vi "Preprocess Action.vi"(0 "Image Type":T2 items=["Grayscale (U8)", "Grayscale (I16)", "Grayscale (SGL)", "Complex (CSG)", "RGB (U32)", "HSL (U32)", "RGB (U64)", "Grayscale (U16)"], 1 "Image Dust":string, 5 "ImageSorce":string, 9 "PreProcess":T1, 11 "error in (no error)":errorcluster, 12 "Data":string) -> (4 "Refnum out":T3, 15 "error out":errorcluster)   [LabVIEW 2019]
uses:
  <vilib>/vision/Image Controls.llb/IMAQ Image.ctl
  Ctrl/VisionProcessName.ctl
  Controls/Process_Setting.ctl
  Controls/CameraAttribute.ctl
  Controls/ProcessBrightness.ctl
  Controls/ExtractPlanParam_Type.ctl
  Controls/ProcessColorThreshold.ctl
  Controls/LookupTableParam.ctl
  Controls/BinaryMonoParam_Type.ctl
  7215dd0e-a700-4e2b-943e-45d7582282bd.vi
  38a9804b-11bb-4e90-8cf5-6f7932444913.vi
  4fbe3eb4-3ab0-49f8-8326-0d8c4c82d423.vi
  17e7e0cf-ffba-40d4-8f93-2ae686572284.vi
  f6032967-3aff-41e1-8fb3-f70b6d7b46ba.vi
  79f2a73c-968e-4675-82f3-10344eb773ba.vi
  0b9d5edb-3a18-4d09-8481-e8059829d2ca.vi
  <vilib>/JDP Science/JSONtext/JSON text to Variant.vi
  <resource>/objmgr/imaqdx.rc
  LLB/Message/MsgShowAndLog.lvlib
panel:
  in  "AutoExposure":enum16{"Off", "Once", "Continuous"}(ring)
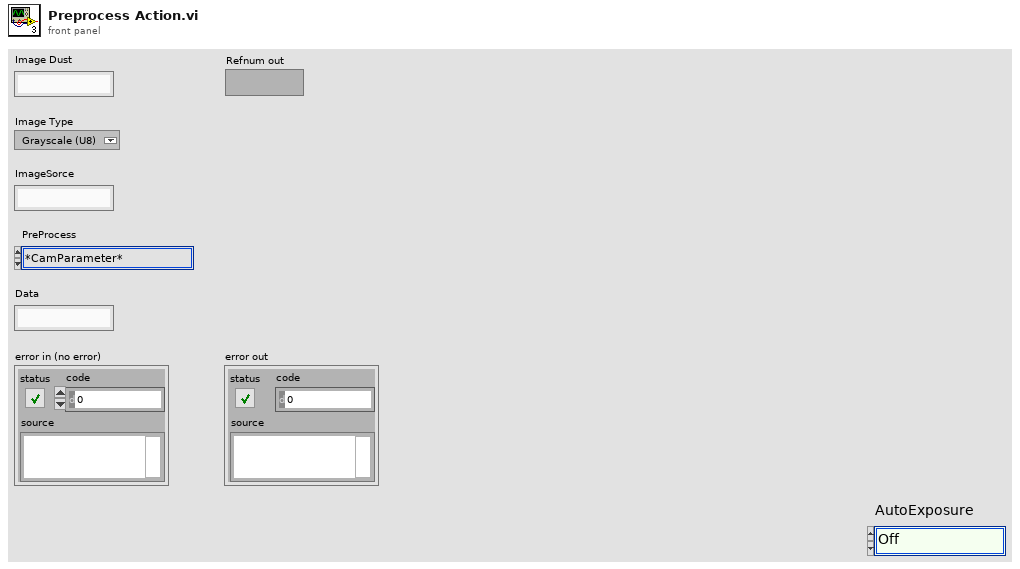
[diagram p1: front panel]
types:
  T1 = typedef "VisionProcessName.ctl" = enum16{"*CamParameter*", "CamAttributes", "*Preprocess*", "CG_Brightness", "C_Plane Extraction", "C_Threshold", "G_Lookup Table", "G_Threshold"}
  T2 = typedef "Image Type" = u32
  T3 = typedef "IMAQ Image.ctl" = refnum<image>
  T4 = typedef "Process_Setting.ctl" = cluster{"Enum_PreProcess":T1, "Parameter":string}
  T5 = enum16{"Init", "Grab", "Get All", "Close", "Set Camera"}
  T6 = typedef "CameraAttribute.ctl" = cluster{"CamName":string, "AutoExposure":enum16{"Off", "Once", "Continuous"}, "Exposure":dbl, "AutoGain":enum16{"Off", "Once", "Continuous"}, "Gain":dbl}
  T7 = typedef "BinaryMonoParam_Type.ctl" = cluster{"Look For":enum16{"Bright Objects", "Dark Objects", "Gray Objects"}, "Threshold":cluster{dbl, dbl}}
  T8 = typedef "IMAQdx.ctl" = refnum<k21>
  T9 = typedef "ProcessBrightness.ctl" = cluster{"Brightness":i32, "Constrast":dbl, "Gamma":dbl}
  T10 = typedef "ExtractPlanParam_Type.ctl" = cluster{"Color Plane":enum16{"Red", "Green", "Blue", "Hue", "Saturation", "Luminance", "Value", "Intensity"}}
  T11 = enum16{"Red", "Green", "Blue", "Hue", "Saturation", "Luminance", "Value", "Intensity"}
  T12 = typedef "ProcessColorThreshold.ctl" = cluster{"Color Mode":u16, "Red or Hue Range":cluster{dbl, dbl}, "Green or Sat Range":cluster{dbl, dbl}, "Blue or Luma or Val or Inten Range":cluster{dbl, dbl}}
  T13 = typedef "LookupTableParam.ctl" = cluster{"Function":enum16{"Equalizer", "Reverse", "Logarithmic", "Exponential", "Square", "Square Root", "Power X", "Power 1/X"}, "Power Value":sgl}
  T14 = enum16{"Equalizer", "Reverse", "Logarithmic", "Exponential", "Square", "Square Root", "Power X", "Power 1/X"}
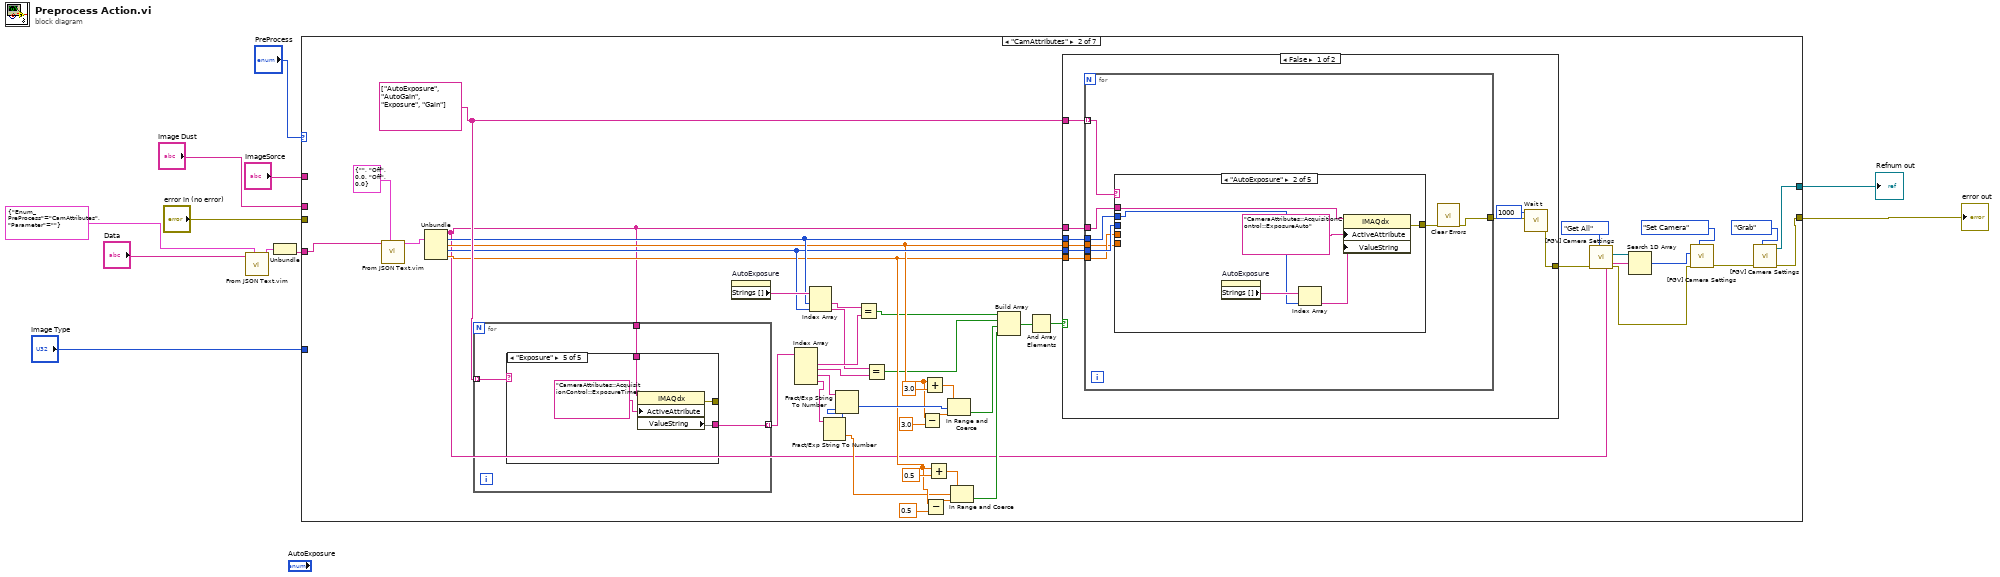
[diagram p0: block diagram]
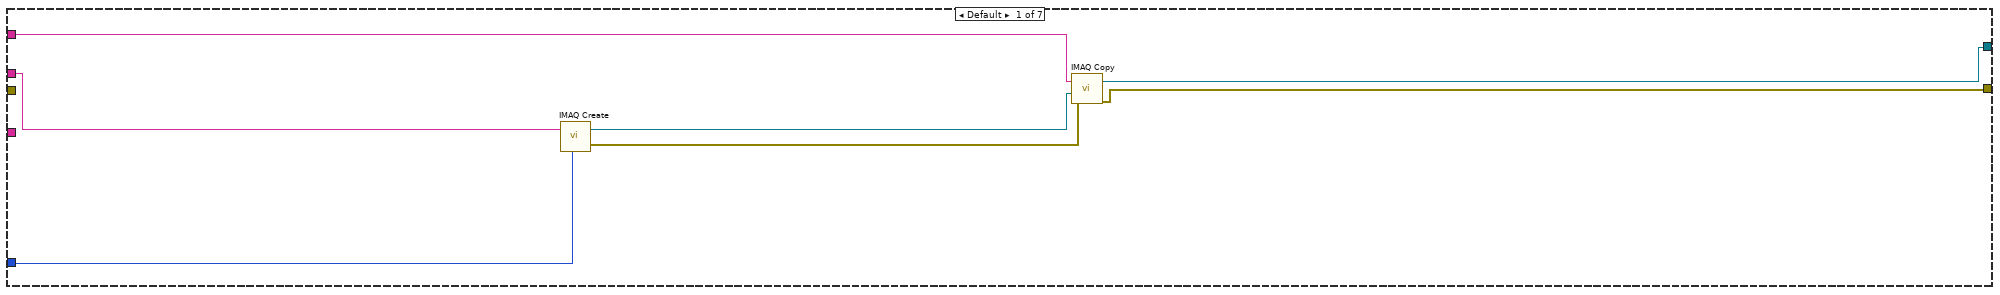
[diagram p2: hidden frame]
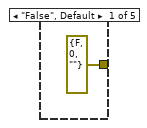
[diagram p3: hidden frame]
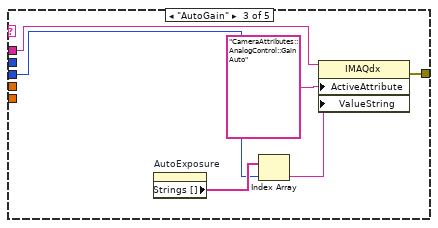
[diagram p4: hidden frame]
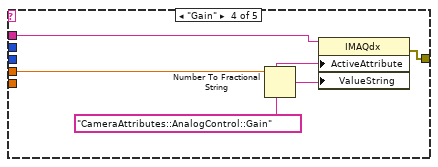
[diagram p5: hidden frame]
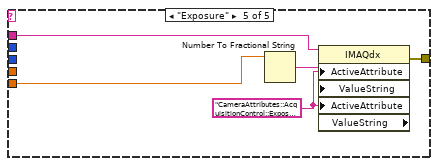
[diagram p6: hidden frame]
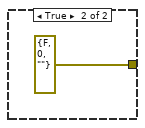
[diagram p7: hidden frame]
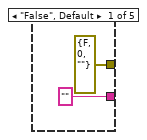
[diagram p8: hidden frame]
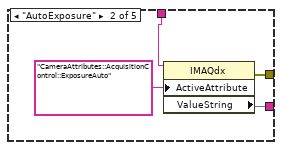
[diagram p9: hidden frame]
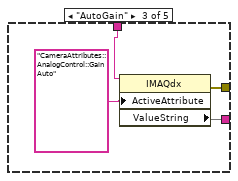
[diagram p10: hidden frame]
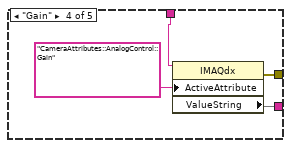
[diagram p11: hidden frame]
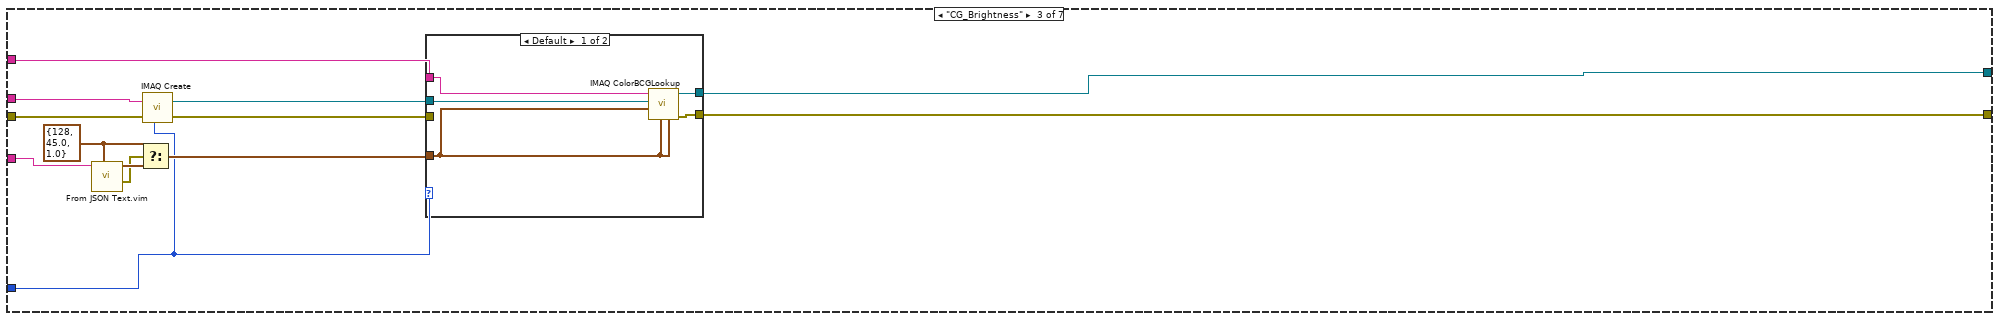
[diagram p12: hidden frame]
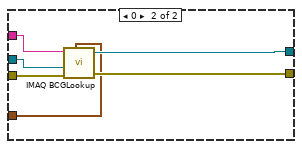
[diagram p13: hidden frame]
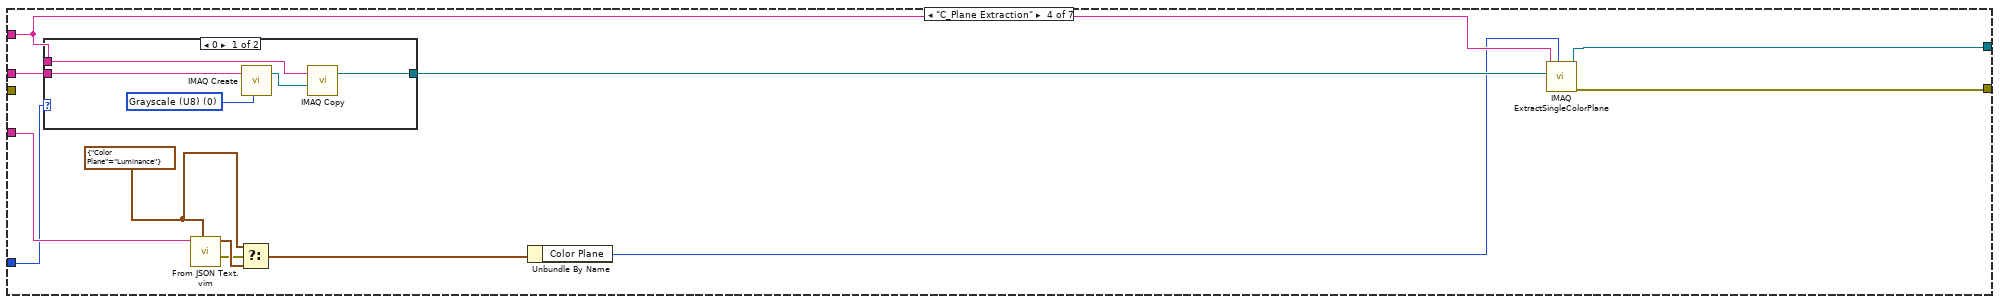
[diagram p14: hidden frame]
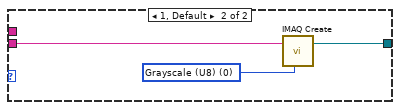
[diagram p15: hidden frame]
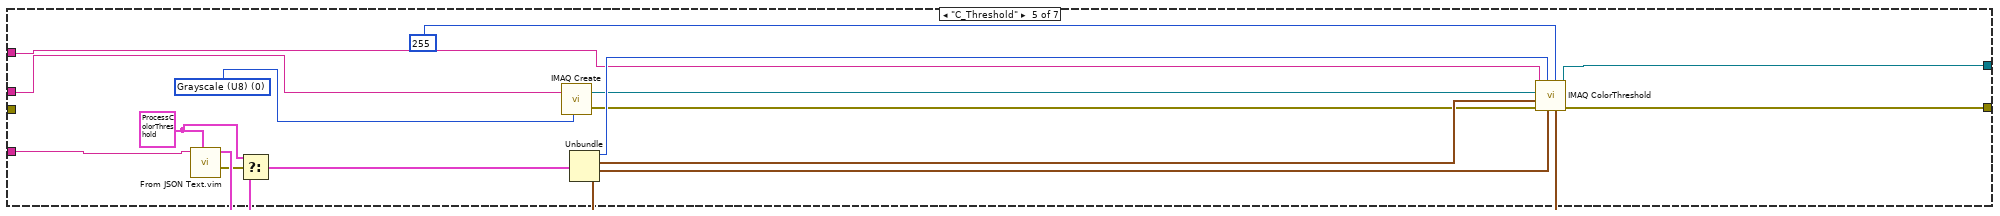
[diagram p16: hidden frame]
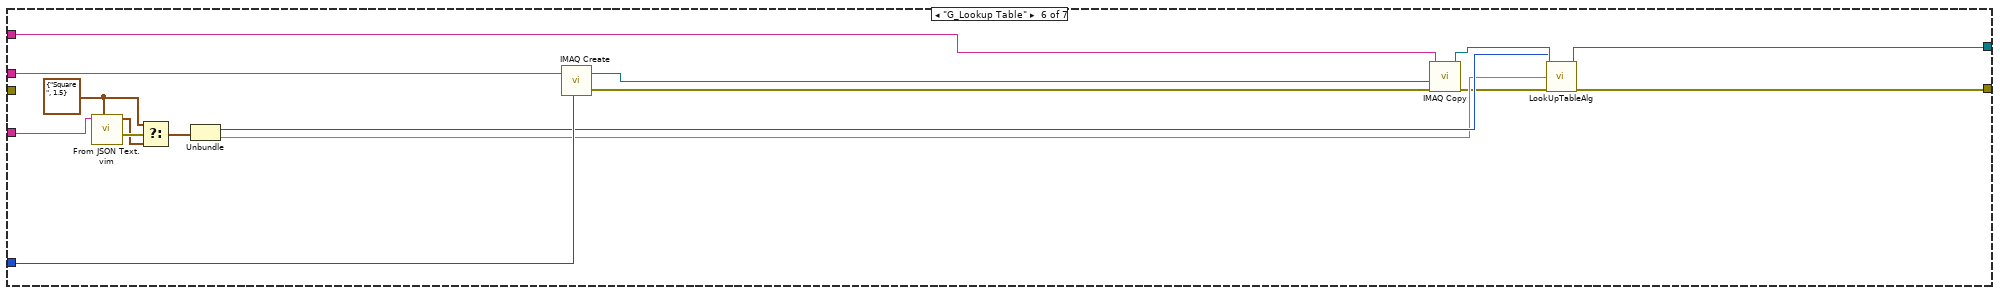
[diagram p17: hidden frame]
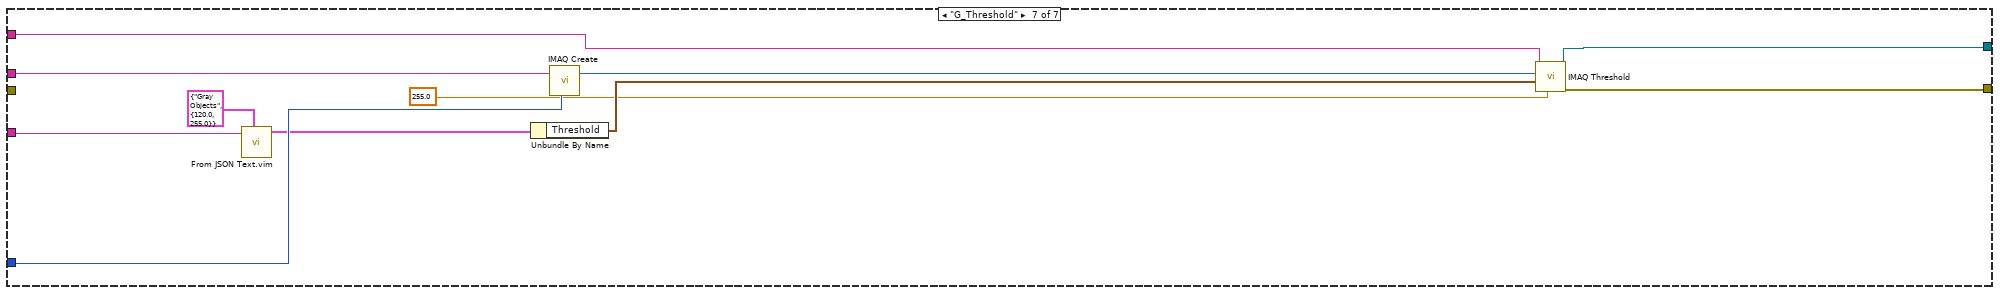
[diagram p18: hidden frame]
diagram:
  n1 = call "From JSON Text.vim"("Data Type and Default Value"=T4 {"Enum_PreProcess"=enum."CamAttributes", "Parameter"=""} ("ProcessSetting"), "JSON"="Data") -> ("Data out"=w3:T4)  [unwired: 8 in, 1 out]
  n2 = Unbundle(w3) -> ("Parameter"=w2:string)  [unwired: 1 out]
  n3 = case shown="\"CamAttributes\"" "PreProcess" {
    tunnel: "Image Type" -> [w18 _ w125 w156 _ w200 w209]
    tunnel: "error in (no error)" -> [_ _ w137 _ _ _ _]
    tunnel: "Image Dust" -> [w17 _ w136 w155 w181 w201 w211]
    tunnel: [w14 w50 w135 w149 w174 w192 w204] -> w9
    tunnel: [w13 w51 w133 w150 w173 w193 w203] -> w10
    tunnel: w2 -> [_ w60 w129 w157 w182 w190 w210]
    tunnel: "ImageSorce" -> [w16 _ w126 w154 w171 w199 w208]
    frame Default {
      n4 = call "IMAQ Create"("Image Name"=w17, "Image Type"=w18) -> ("New Image"=w15:T3, "error out"=w12:errorcluster)  [unwired: 3 in]
      n5 = call "IMAQ Copy"("error in (no error)"=w12, "Image Dst"=w15, "Image Src"=w16) -> ("error out"=w13:errorcluster, "Image Dst Out"=w14:T3)  [unwired: 3 in]
    }
    frame "CamAttributes" {
      w49 = string[] ["AutoExposure", "AutoGain", "Exposure", "Gain"]
      n6 = call "From JSON Text.vim"("Data Type and Default Value"=T6 {"CamName"="", "AutoExposure"=enum."Off", "Exposure"=0.0, "AutoGain"=enum."Off", "Gain"=0.0} ("CamAttribute"), "JSON"=w60) -> ("Data out"=w61:T6)  [unwired: 8 in, 1 out]
      n7 = Unbundle(w61) -> ("CamName"=w21:string, "AutoExposure"=w47:enum16{"Off", "Once", "Continuous"}, "Exposure"=w37:dbl, "AutoGain"=w46:enum16{"Off", "Once", "Continuous"}, "Gain"=w31:dbl)
      n8 = for {
        tunnel: w49 -> [w106] mode=indexing
        tunnel: [w105] -> w44 mode=indexing
        tunnel: w21 -> [w104]
        n9 = case shown="\"Exposure\"" w106 {
          tunnel: [errorcluster {"status"=FALSE, "code"=0, "source"=""} ("error out") w111 w115 w119 w123] -> _
          tunnel: ["" ("ValueString") w110 w114 w118 w122] -> w105
          tunnel: w104 -> [_ w109 w113 w117 w121]
          frame "False", Default {
          }
          frame "AutoExposure" {
            n10 = property class="IMAQdx"(reference=w109, "ActiveAttribute"="CameraAttributes::AcquisitionControl::ExposureAuto") -> (error out=w111:errorcluster, "ValueString"=w110)  [unwired: 1 in, 1 out]
          }
          frame "AutoGain" {
            n11 = property class="IMAQdx"(reference=w113, "ActiveAttribute"="CameraAttributes::AnalogControl::GainAuto") -> (error out=w115:errorcluster, "ValueString"=w114)  [unwired: 1 in, 1 out]
          }
          frame "Gain" {
            n12 = property class="IMAQdx"(reference=w117, "ActiveAttribute"="CameraAttributes::AnalogControl::Gain") -> (error out=w119:errorcluster, "ValueString"=w118)  [unwired: 1 in, 1 out]
          }
          frame "Exposure" {
            n13 = property class="IMAQdx"(reference=w121, "ActiveAttribute"="CameraAttributes::AcquisitionControl::ExposureTime") -> (error out=w123:errorcluster, "ValueString"=w122)  [unwired: 1 in, 1 out]
          }
        }
      }
      n14 = property on="AutoExposure" class="Enum (strict)"() -> ("Strings []"=w48:string[])  [unwired: 2 in, 2 out]
      n15 = Index Array(array=w44) -> (element #1=w43:string, element #2=w20:string, element #3=w19:string, element #4=w29:string)  [unwired: 4 in]
      n16 = Index Array(array=w48, index #1=w47, index #2=w46) -> (element #1=w45:string, element #2=w42:string)
      n17 = Fract/Exp String To Number(string=w29) -> (offset past number=w30:i32, number=w28:dbl)  [unwired: 3 in]
      n18 = Fract/Exp String To Number(string=w19, default (0 dbl)=w30) -> (number=w41:i32)  [unwired: 2 in, 1 out]
      n19 = Equal?(x=w45, y=w43) -> (x = y?=w27:bool)
      n20 = Equal?(x=w42, y=w20) -> (x = y?=w26:bool)
      n21 = Subtract(x=w37, y=3.0) -> (x-y=w38:dbl)
      n22 = Add(x=w37, y=3.0) -> (x+y=w40:dbl)
      n23 = Subtract(x=w31, y=0.5) -> (x-y=w34:dbl)
      n24 = Add(x=w31, y=0.5) -> (x+y=w32:dbl)
      n25 = In Range and Coerce(upper limit=w40, x=w41, lower limit=w38) -> (In Range?=w25:bool)  [unwired: 1 out]
      n26 = In Range and Coerce(upper limit=w32, x=w28, lower limit=w34) -> (In Range?=w24:bool)  [unwired: 1 out]
      n27 = Build Array(w27, w26, w25, w24) -> (w23:bool[])
      n28 = And Array Elements(Boolean array=w23) -> (logical AND=w22:bool)
      n29 = case shown="False" w22 {
        tunnel: w21 -> [w71 _]
        tunnel: [w64 errorcluster {"status"=FALSE, "code"=0, "source"=""} ("error out")] -> w52
        tunnel: w49 -> [w69 _]
        tunnel: w47 -> [w68 _]
        tunnel: w46 -> [w67 _]
        tunnel: w37 -> [w66 _]
        tunnel: w31 -> [w65 _]
        frame False {
          n30 = for {
            tunnel: w69 -> [w72] mode=indexing
            tunnel: w68 -> [w79]
            tunnel: w71 -> [w78]
            tunnel: [w75] -> w70
            tunnel: w67 -> [w77]
            tunnel: w65 -> [w74]
            tunnel: w66 -> [w73]
            n31 = case shown="\"AutoExposure\"" w72 {
              tunnel: w79 -> [_ w84 _ _ _]
              tunnel: w78 -> [_ w83 w91 w93 w100]
              tunnel: w77 -> [_ _ w89 _ _]
              tunnel: [errorcluster {"status"=FALSE, "code"=0, "source"=""} ("error out") w81 w87 w94 w98] -> w76
              tunnel: w74 -> [_ _ _ w95 _]
              tunnel: w73 -> [_ _ _ _ w99]
              frame "False", Default {
              }
              frame "AutoExposure" {
                n32 = property on="AutoExposure" class="Enum (strict)"() -> ("Strings []"=w85:string[])  [unwired: 2 in, 2 out]
                n33 = Index Array(array=w85, index=w84) -> (element=w82:string)
                n34 = property class="IMAQdx"(reference=w83, "ActiveAttribute"="CameraAttributes::AcquisitionControl::ExposureAuto", "ValueString"=w82) -> (error out=w81:errorcluster)  [unwired: 1 in, 1 out]
              }
              frame "AutoGain" {
                n35 = property on="AutoExposure" class="Enum (strict)"() -> ("Strings []"=w90:string[])  [unwired: 2 in, 2 out]
                n36 = Index Array(array=w90, index=w89) -> (element=w88:string)
                n37 = property class="IMAQdx"(reference=w91, "ActiveAttribute"="CameraAttributes::AnalogControl::GainAuto", "ValueString"=w88) -> (error out=w87:errorcluster)  [unwired: 1 in, 1 out]
              }
              frame "Gain" {
                n38 = Number To Fractional String(number=w95) -> (F-format string=w96:string)  [unwired: 3 in]
                n39 = property class="IMAQdx"(reference=w93, "ActiveAttribute"="CameraAttributes::AnalogControl::Gain", "ValueString"=w96) -> (error out=w94:errorcluster)  [unwired: 1 in, 1 out]
              }
              frame "Exposure" {
                w102 = "CameraAttributes::AcquisitionControl::ExposureTime" ("ActiveAttribute")
                n40 = Number To Fractional String(number=w99) -> (F-format string=w101:string)  [unwired: 3 in]
                n41 = property class="IMAQdx" props=["ActiveAttribute", "ValueString", "ActiveAttribute", "ValueString"](reference=w100, "ActiveAttribute"=w102, "ValueString"=w101, "ActiveAttribute"=w102) -> (error out=w98:errorcluster)  [unwired: 1 in, 2 out]
              }
            }
            n42 = call <vilib>:"Clear Errors.vi"("error in (no error)"=w76) -> ("error out"=w75:errorcluster)  [unwired: 5 in, 1 out]
          }
          n43 = call "Wait t.vi"("error in"=w70, "wait(ms)"=u32 1000) -> ("error out"=w64:errorcluster)  [unwired: 9 in]
        }
        frame True {
        }
      }
      n44 = call "[FGV] Camera Settings.vi"("Action"=T5."Get All", "error in (no error)"=w52) -> ("error out"=w55:errorcluster, "Camera Interface Name"=w58:T8[])  [unwired: 7 in, 1 out]
      n45 = Search 1D Array(1D array=w58, element=w21) -> (index of element=w56:i32)  [unwired: 1 in]
      n46 = call "[FGV] Camera Settings.vi"("Action"=T5."Set Camera", "error in (no error)"=w55, "Value"=w56) -> ("error out"=w53:errorcluster)  [unwired: 6 in, 2 out]
      n47 = call "[FGV] Camera Settings.vi"("Action"=T5."Grab", "error in (no error)"=w53) -> ("error out"=w51:errorcluster, "Image Out"=w50:T3)  [unwired: 7 in, 1 out]
    }
    frame "CG_Brightness" {
      w132 = T9 {"Brightness"=128, "Constrast"=45.0, "Gamma"=1.0} ("t")
      n48 = call "From JSON Text.vim"("Data Type and Default Value"=w132, "JSON"=w129) -> ("error out"=w130:errorcluster, "Data out"=w131:T9)  [unwired: 8 in]
      n49 = Select(t=w132, s=w130, f=w131) -> (s? t:f=w128:T9)
      n50 = call "IMAQ Create"("Image Name"=w136, "Image Type"=w125, "error in (no error)"=w137) -> ("New Image"=w127:T3, "error out"=w134:errorcluster)  [unwired: 2 in]
      n51 = case shown="Default" w125 {
        tunnel: [w138 w148] -> w135
        tunnel: w134 -> [_ w147]
        tunnel: [w139 w146] -> w133
        tunnel: w128 -> [w140 w145]
        tunnel: w127 -> [w141 w144]
        tunnel: w126 -> [w142 w143]
        frame Default {
          n52 = call "IMAQ ColorBCGLookup"("Blue BCG Values"=w140, "Green BCG Values"=w140, "Red BCG Values"=w140, "Image Dst"=w141, "Image Src"=w142) -> ("error out"=w139:errorcluster, "Image Dst Out"=w138:T3)  [unwired: 2 in, 3 out]
        }
        frame 0 {
          n53 = call "IMAQ BCGLookup"("Image Src"=w143, "BCG Values"=w145, "Image Dst"=w144, "error in (no error)"=w147) -> ("Image Dst Out"=w148:T3, "error out"=w146:errorcluster)  [unwired: 1 in, 2 out]
        }
      }
    }
    frame "C_Plane Extraction" {
      w160 = T10 {"Color Plane"=enum."Luminance"} ("ExtractPlanParam")
      n54 = case shown="0" w156 {
        tunnel: w155 -> [w165 w168]
        tunnel: w154 -> [w162 _]
        tunnel: [w161 w166] -> w153
        frame 0 {
          w164 = T2 0 items=["Grayscale (U8)", "Grayscale (I16)", "Grayscale (SGL)", "Complex (CSG)", "RGB (U32)", "HSL (U32)", "RGB (U64)", "Grayscale (U16)"] ("Image Type")
          n55 = call "IMAQ Create"("Image Name"=w165, "Image Type"=w164) -> ("New Image"=w163:T3)  [unwired: 3 in, 1 out]
          n56 = call "IMAQ Copy"("Image Dst"=w163, "Image Src"=w162) -> ("Image Dst Out"=w161:T3)  [unwired: 4 in, 1 out]
        }
        frame 1, Default {
          w167 = T2 0 items=["Grayscale (U8)", "Grayscale (I16)", "Grayscale (SGL)", "Complex (CSG)", "RGB (U32)", "HSL (U32)", "RGB (U64)", "Grayscale (U16)"] ("Image Type")
          n57 = call "IMAQ Create"("Image Name"=w168, "Image Type"=w167) -> ("New Image"=w166:T3)  [unwired: 3 in, 1 out]
        }
      }
      n58 = call "From JSON Text.vim"("Data Type and Default Value"=w160, "JSON"=w157) -> ("error out"=w158:errorcluster, "Data out"=w159:T10)  [unwired: 8 in]
      n59 = Select(t=w160, s=w158, f=w159) -> (s? t:f=w152:T10)
      n60 = Unbundle By Name(w152) -> ("Color Plane"=w151:T11)
      n61 = call "IMAQ ExtractSingleColorPlane"("Color Plane"=w151, "Image Dst"=w153, "Image Src"=w154) -> ("error out"=w150:errorcluster, "Image Dst Out"=w149:T3)  [unwired: 7 in]
    }
    frame "C_Threshold" {
      w169 = T2 0 items=["Grayscale (U8)", "Grayscale (I16)", "Grayscale (SGL)", "Complex (CSG)", "RGB (U32)", "HSL (U32)", "RGB (U64)", "Grayscale (U16)"] ("Image Type")
      w184 = T12 {"Color Mode"=0, "Red or Hue Range"={120.0, 255.0}, "Green or Sat Range"={120.0, 255.0}, "Blue or Luma or Val or Inten Range"={120.0, 255.0}} ("ColorThreshold")
      n62 = call "From JSON Text.vim"("Data Type and Default Value"=w184, "JSON"=w182) -> ("error out"=w183:errorcluster, "Data out"=w185:T12)  [unwired: 8 in]
      n63 = Select(t=w184, s=w183, f=w185) -> (s? t:f=w180:T12)
      n64 = call "IMAQ Create"("Image Name"=w181, "Image Type"=w169) -> ("New Image"=w170:T3, "error out"=w172:errorcluster)  [unwired: 3 in]
      n65 = Unbundle(w180) -> ("Color Mode"=w176:u16, "Red or Hue Range"=w179:cluster{dbl, dbl}, "Green or Sat Range"=w178:cluster{dbl, dbl}, "Blue or Luma or Val or Inten Range"=w177:cluster{dbl, dbl})
      n66 = call "IMAQ ColorThreshold"("Blue or Luma or Val or Inten Range"=w177, "Replace Value"=255, "Green or Sat Range"=w178, "Color Mode"=w176, "error in (no error)"=w172, "Red or Hue Range"=w179, "Image Dst"=w170, "Image Src"=w171) -> ("error out"=w173:errorcluster, "Image Dst Out"=w174:T3)  [unwired: 2 in]
    }
    frame "G_Lookup Table" {
      w186 = T13 {"Function"=enum."Square", "Power Value"=1.5} ("LookupTableParam")
      n67 = call "From JSON Text.vim"("Data Type and Default Value"=w186, "JSON"=w190) -> ("error out"=w188:errorcluster, "Data out"=w187:T13)  [unwired: 8 in]
      n68 = Select(t=w186, s=w188, f=w187) -> (s? t:f=w189:T13)
      n69 = Unbundle(w189) -> ("Function"=w195:T14, "Power Value"=w194:sgl)
      n70 = call "IMAQ Create"("Image Name"=w201, "Image Type"=w200) -> ("New Image"=w198:T3, "error out"=w197:errorcluster)  [unwired: 3 in]
      n71 = call "IMAQ Copy"("error in (no error)"=w197, "Image Dst"=w198, "Image Src"=w199) -> ("error out"=w191:errorcluster, "Image Dst Out"=w196:T3)  [unwired: 3 in]
      n72 = call "LookUpTableAlg.vi"("ImageIn"=w196, "Function"=w195, "Power Value"=w194, "error In"=w191) -> ("Image Dst Out"=w192:T3, "error out"=w193:errorcluster)  [unwired: 10 in]
    }
    frame "G_Threshold" {
      n73 = call "From JSON Text.vim"("Data Type and Default Value"=T7 {"Look For"=enum."Gray Objects", "Threshold"={120.0, 255.0}} ("MonoThreshold"), "JSON"=w210) -> ("Data out"=w206:T7)  [unwired: 8 in, 1 out]
      n74 = Unbundle By Name(w206) -> ("Threshold"=w205:cluster{dbl, dbl})
      n75 = call "IMAQ Create"("Image Name"=w211, "Image Type"=w209) -> ("New Image"=w207:T3)  [unwired: 3 in, 1 out]
      n76 = call "IMAQ Threshold"("Replace Value"=sgl 255.0, "Range"=w205, "Image Dst"=w207, "Image Src"=w208) -> ("error out"=w203:errorcluster, "Image Dst Out"=w204:T3)  [unwired: 6 in]
    }
  }
  "error out" <- w10
  "Refnum out" <- w9
